vi "sensor value make from realnum.vi"(6 "formatter":string, 7 "unit":string, 8 "error in (no error)":errorcluster, 9 "value":dbl, 10 "name":string, 11 "h":u64) -> (0 "error out":errorcluster, 2 "function return":u32(ring), 3 "h out":u64)   [LabVIEW 2023, in "uhd.lvlib"]
doc: "UHD_API uhd_error uhd_sensor_value_make_from_realnum(uhd_sensor_value_handle* h,\n const char* name,\n double value,\n const char* unit,\n const char* formatter);"
uses:
  <userlib>/uhd/uhd.lvlib
  <userlib>/uhd/uhd.dll
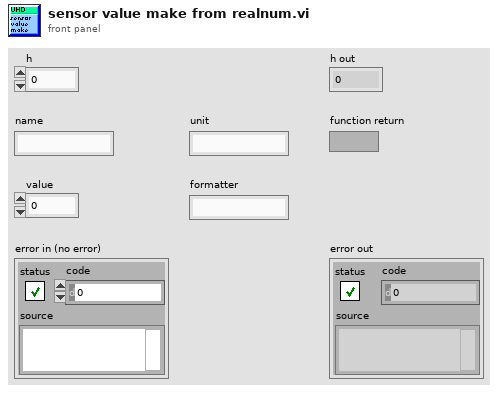
[diagram p1: front panel]
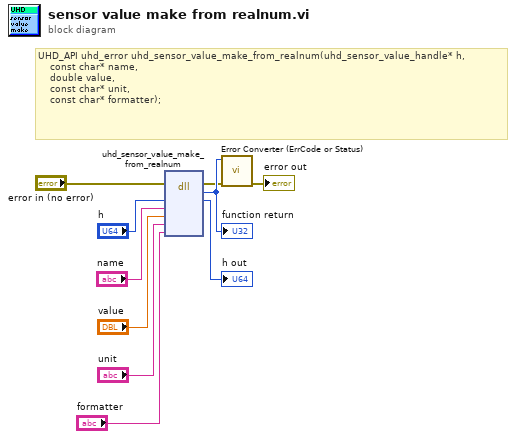
[diagram p0: block diagram]
diagram:
  # "UHD_API uhd_error uhd_sensor_value_make_from_realnum(uhd_sensor_value_handle* h,\n    const char* name,\n    double value,\n    const char* unit,\n    const char* formatter);"
  n1 = dll-call lib="C:/Program Files/National Instruments/LabVIEW 2023/user.lib/uhd/uhd.*" fn="uhd_sensor_value_make_from_realnum"(error in="error in (no error)", "h"="h", "name"="name", "value"="value", "unit"="unit", "formatter"="formatter") -> (error out=w2:errorcluster, w10:u32, "h"=→"h out":u64)  [unwired: 6 in, 1 out]
  "function return" <- w10
  n2 = call <userlib>:"Error Converter (ErrCode or Status).vi"("error in (no error)"=w2, "error code"=w10) -> ("error out"=→"error out":errorcluster)  [unwired: 9 in]
